vi "PathPlanner_RotationTarget_GetPosition.vi"(11 "RotationTarget":T1={"rotation"={"VALUE"=0.0, "COS"=1.0, "SIN"=0.0}, "position"=0.0, "Exists"=FALSE} {"rotation"."SIN" format="%13.4f"; "rotation"."COS" format="%13.4f"; "rotation"."VALUE" format="%13.4f"}) -> (0 "Exists":bool, 3 "position":dbl)   [LabVIEW 2019, in "PathPlanner24.lvlib"]
doc: "Get data elements of a rotation target. \n\nInputs: \n - RotationTarget - cluster - defined rotation target data structure\n \nOutputs:\n - position - double - Waypoint relative position of this target\n - rotation - rotation2d - Target rotation\n - exists - boolean - TRUE if not null - Exists - boolean - TRUE if rotation target is not null"
uses:
  TypeDef/PathPlannerRotationTarget.ctl
  <vilib>/Rock Robotics/WPI/ThirdParty/JAS_Junk/TrajLib/TypeDef/ROTATION2D.ctl
  PathPlanner24.lvlib
  <vilib>/Rock Robotics/WPI/ThirdParty/JAS_Junk/TrajLib/Trajectory_Library.lvlib
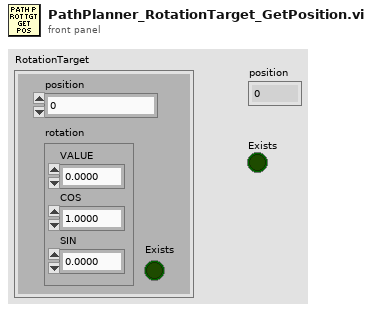
[diagram p1: front panel]
types:
  T1 = typedef "PathPlanner24.lvlib/PathPlannerRotationTarget.ctl" = cluster{"rotation":T2, "position":dbl, "Exists":bool}
  T2 = typedef "Trajectory_Library.lvlib/ROTATION2D.ctl" = cluster{"VALUE":dbl, "COS":dbl, "SIN":dbl}
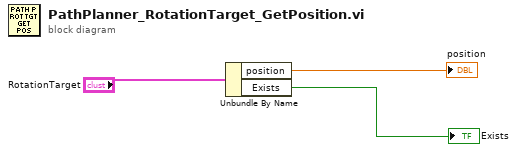
[diagram p0: block diagram]
diagram:
  n1 = Unbundle By Name("RotationTarget") -> ("position"=→"position":dbl, "Exists"=→"Exists":bool)
